vi "Periodic Tasks.vi"(8 "error in":errorcluster) -> ()   [LabVIEW 2018]
doc: "This VI runs in parallel to other tasks. It can contain as many user-defined periodic loops as you need. These can carry out PID or other sorts of timed response."
uses:
  <vilib>/Rock Robotics/WPI/Solenoid/WPI_SolenoidValue.ctl
  Robot Global Data.vi
  <vilib>/Rock Robotics/WPI/Solenoid/WPI_SolenoidSetEnum.vi
  <vilib>/Rock Robotics/Network Tables/NT Read Number.vi
panel:
  out "error out":errorcluster
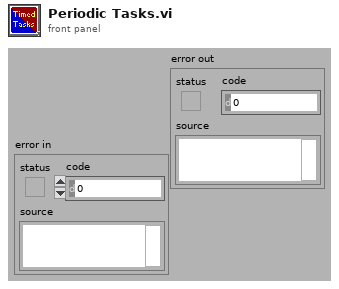
[diagram p1: front panel]
types:
  T1 = typedef "WPI_SolenoidValue.ctl" = enum16{"Off", "On", "Forward", "Reverse"}
  T2 = typedef "WPI_SolenoidDevRef.ctl" = cluster{"DevStatus":errorcluster, "Pneumatics Control Module":u8, "Forward Solenoid Channel":T3, "Reverse Solenoid Channel":T3}
  T3 = typedef "WPI_SolenoidChannel.ctl" = enum8{"Solenoid 0", "Solenoid 1", "Solenoid 2", "Solenoid 3", "Solenoid 4", "Solenoid 5", "Solenoid 6", "Solenoid 7", "Invalid"}
  T4 = cluster{"offsetAngle H":dbl, "offsetAngle V":dbl, "area":dbl, "skew":dbl}
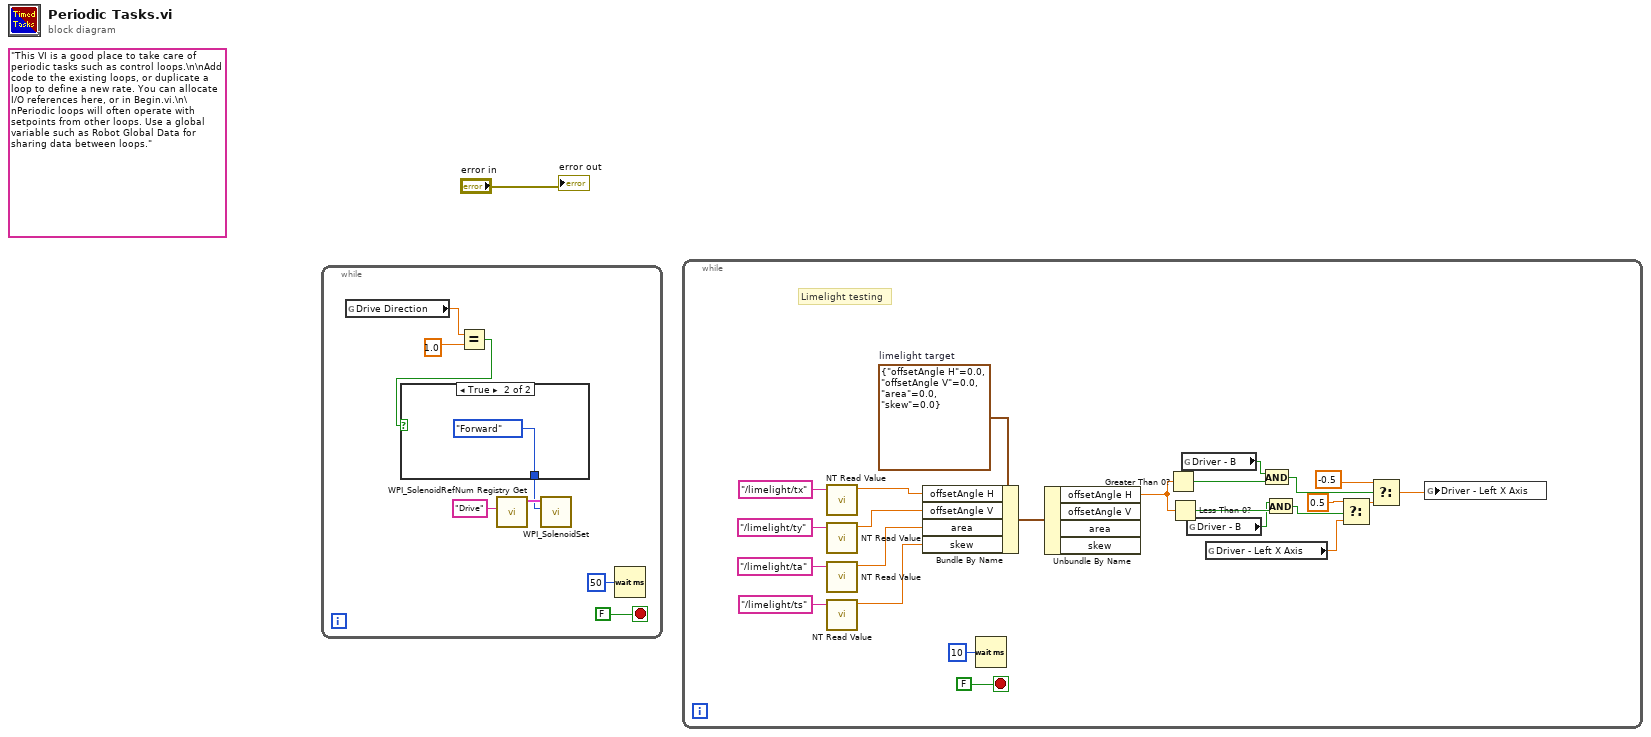
[diagram p0: block diagram]
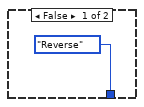
[diagram p2: hidden frame]
diagram:
  (unwired) "This VI is a good place to take care of periodic tasks such as control loops.\n\nAdd code to the existing loops, or duplicate a loop to define a new rate. You can allocate I/O references here, or in Begin.vi.\n\nPeriodic loops will often operate with setpoints from other loops. Use a global variable such as Robot Global Data for sharing data between loops."
  n1 = while {
    stop <- FALSE stop-if-true
    n2 = global read "Robot Global Data.vi" "Drive Direction"() -> (w6:dbl)
    n3 = Equal?(x=w6, y=1.0) -> (x = y?=w5:bool)
    n4 = case shown="True" w5 {
      tunnel: [WPI_SolenoidValue."Reverse" ("Value") WPI_SolenoidValue."Forward" ("Value")] -> w2
      frame False {
      }
      frame True {
      }
    }
    n5 = call <vilib>:"WPI_SolenoidRefNum Registry Get.vi"("refnum name"="Drive") -> ("SolenoidDevRef"=w4:T2)  [unwired: 9 in, 1 out]
    n6 = call-poly <vilib>:"WPI_SolenoidSet.vi"("Value"=w2, "SolenoidDevRef"=w4) -> ()  [unwired: 8 in, 2 out]
    n7 = Wait (ms)(milliseconds to wait=u32 50) -> ()  [unwired: 1 out]
  }
  n8 = while {
    stop <- FALSE stop-if-true
    w25 = T4 {"offsetAngle H"=0.0, "offsetAngle V"=0.0, "area"=0.0, "skew"=0.0}  # limelight target
    # "Limelight testing"
    n9 = call-poly <vilib>:"NT Read Value.vi"("Name"="/limelight/tx") -> ("Numeric"=w26:dbl)  [unwired: 9 in, 1 out]
    n10 = call-poly <vilib>:"NT Read Value.vi"("Name"="/limelight/ty") -> ("Numeric"=w27:dbl)  [unwired: 9 in, 1 out]
    n11 = call-poly <vilib>:"NT Read Value.vi"("Name"="/limelight/ta") -> ("Numeric"=w28:dbl)  [unwired: 9 in, 1 out]
    n12 = call-poly <vilib>:"NT Read Value.vi"("Name"="/limelight/ts") -> ("Numeric"=w29:dbl)  [unwired: 9 in, 1 out]
    n13 = Bundle By Name(cluster=w25, "offsetAngle H"=w26, "offsetAngle V"=w27, "area"=w28, "skew"=w29) -> (w30:T4)
    n14 = Wait (ms)(milliseconds to wait=u32 10) -> ()  [unwired: 1 out]
    n15 = Unbundle By Name(w30) -> ("offsetAngle H"=w18:dbl)  [unwired: 3 out]
    n16 = Greater Than 0?(x=w18) -> (x > 0?=w31:bool)
    n17 = Less Than 0?(x=w18) -> (x < 0?=w17:bool)
    n18 = global read "Robot Global Data.vi" "Driver - B"() -> (w32:bool)
    n19 = global read "Robot Global Data.vi" "Driver - B"() -> (w16:bool)
    n20 = global read "Robot Global Data.vi" "Driver - Left X Axis"() -> (w12:dbl)
    n21 = And(x=w32, y=w31) -> (x .and. y?=w33:bool)
    n22 = And(x=w16, y=w17) -> (x .and. y?=w15:bool)
    n23 = Select(t=0.5 ("y"), s=w15, f=w12) -> (s? t:f=w13:dbl)
    n24 = Select(t=-0.5 ("y"), s=w33, f=w13) -> (s? t:f=w19:dbl)
    n25 = global write "Robot Global Data.vi" "Driver - Left X Axis"(w19) -> ()
  }
  "error out" <- "error in"
